vi "Find Cal State.vi"(0 "TrackingSection":string[][](array[string])) -> (4 "StateArray":i32[](array[numeric]), 8 "EnabledStates":bool[](array[boolean]), 15 "CurrentState":i32)   [LabVIEW 2013]
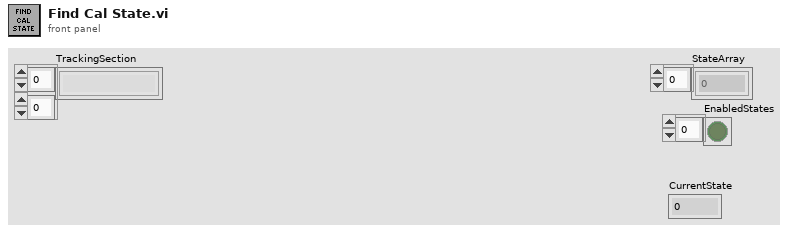
[diagram p1: front panel]
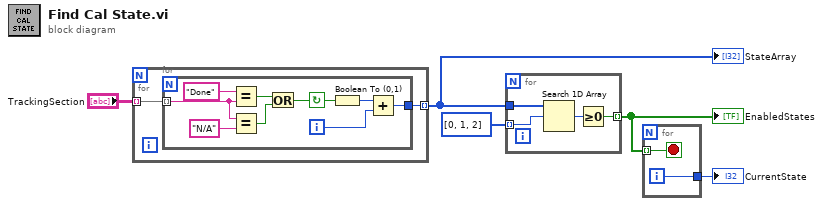
[diagram p0: block diagram]
diagram:
  n1 = for {
    tunnel: "TrackingSection" -> [w7] mode=indexing
    tunnel: [w6] -> w4 mode=indexing
    n2 = for {
      tunnel: w7 -> [w16] mode=indexing
      tunnel: [w8] -> w6
      i -> [w9]
      stop <- w11 continue-if-true
      n3 = Equal?(x="Done", y=w16) -> (x = y?=w13:bool)
      n4 = Equal?(x=w16, y="N/A") -> (x = y?=w12:bool)
      n5 = Or(x=w13, y=w12) -> (x .or. y?=w11:bool)
      n6 = Boolean To (0,1)(Boolean=w11) -> (0, 1=w10:i16)
      n7 = Add(x=w10, y=w9) -> (x+y=w8:i32)
    }
  }
  "StateArray" <- w4
  n8 = for {
    tunnel: w4 -> [w20]
    tunnel: i32[] [0, 1, 2] -> [w19] mode=indexing
    tunnel: [w17] -> w2 mode=indexing
    n9 = Search 1D Array(1D array=w20, element=w19) -> (index of element=w18:i32)  [unwired: 1 in]
    n10 = Greater Or Equal To 0?(x=w18) -> (x >= 0?=w17:bool)
  }
  "EnabledStates" <- w2
  n11 = for {
    tunnel: w2 -> [w22] mode=indexing
    tunnel: [w21] -> w1
    i -> [w21]
    stop <- w22 stop-if-true
  }
  "CurrentState" <- w1
